vi "findfreebuffers.vi"(10 "Buffers":T1[](array[typedef])) -> (2 "unlock buffers":i32)   [LabVIEW 2016]
uses:
  private/vis/BufferStruct.ctl
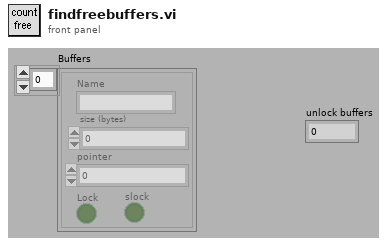
[diagram p1: front panel]
types:
  T1 = typedef "BufferStruct.ctl" = cluster{"Name":string, "size (bytes)":u64, "pointer":u64, "Lock":bool, "slock":bool}
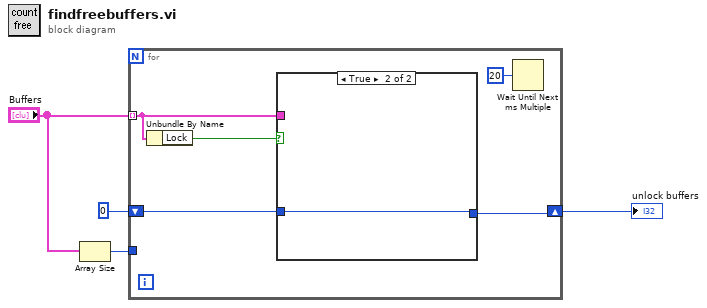
[diagram p0: block diagram]
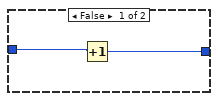
[diagram p2: hidden frame]
diagram:
  n1 = Array Size(array="Buffers") -> (size(s)=w3:i32)
  n2 = for {
    tunnel: "Buffers" -> [w9] mode=indexing
    tunnel: w3 -> [_]
    shift-right: [w6] -> w1
    shift-left: 0 -> [w7]
    n3 = Unbundle By Name(w9) -> ("Lock"=w8:bool)
    n4 = case shown="True" w8 {
      tunnel: w9 -> [_ _]
      tunnel: w7 -> [w11 w12]
      tunnel: [w10 w12] -> w6
      frame False {
        n5 = Increment(x=w11) -> (x+1=w10:i32)
      }
      frame True {
        (unwired) TRUE
      }
    }
    n6 = Wait Until Next ms Multiple(millisecond multiple=u32 20) -> ()  [unwired: 1 out]
  }
  "unlock buffers" <- w1
